vi "Datenauswertung.vi"(7 "Zeit seit dem letzten Aufruf":u32, 8 "Iterationszähler":u8, 11 "Daten aus FPGA-Speicher":u8) -> (0 "Daten für FIFO":u8)   [LabVIEW 2013]
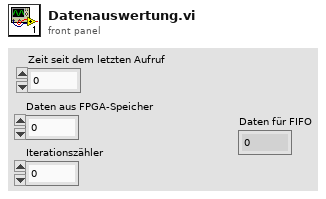
[diagram p1: front panel]
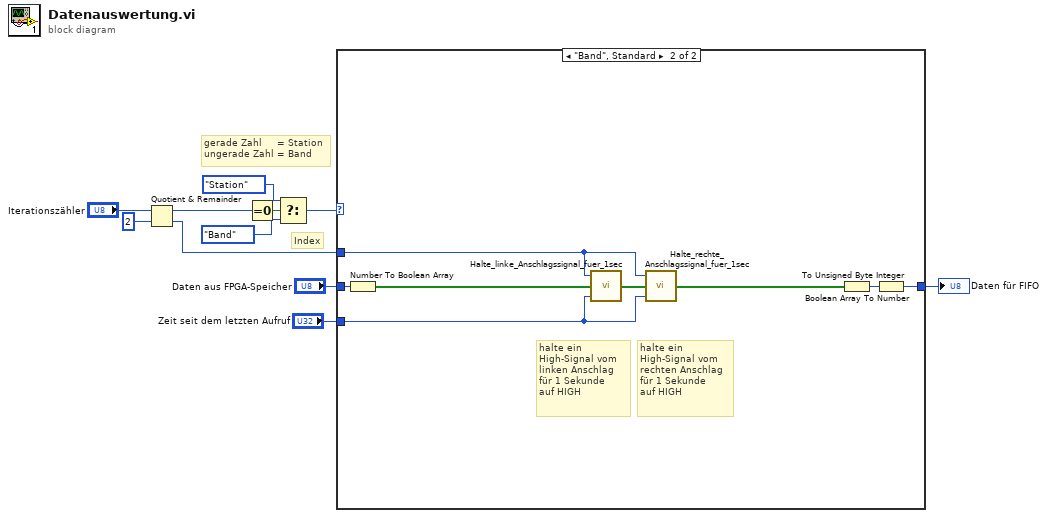
[diagram p0: block diagram]
diagram:
  # "Index"
  # "gerade Zahl     = Station\nungerade Zahl = Band"
  n1 = Quotient & Remainder(x="Iterationszähler", y=u8 2) -> (x-y*floor(x/y)=w5:u8, floor(x/y)=w9:u8)
  n2 = Equal To 0?(x=w5) -> (x = 0?=w4:bool)
  n3 = Select(t=enum16{"Station", "Band"}."Station", s=w4, f=enum16{"Station", "Band"}."Band") -> (s? t:f=w1:enum16{"Station", "Band"})
  n4 = case shown="\"Band\", Standard" w1 {
    tunnel: w9 -> [_ w15]
    tunnel: "Daten aus FPGA-Speicher" -> [w12 w19]
    tunnel: [w12 w13] -> w6
    tunnel: "Zeit seit dem letzten Aufruf" -> [_ w20]
    frame "Station" {
    }
    frame "Band", Default {
      # "halte ein \nHigh-Signal vom\nrechten Anschlag\nfür 1 Sekunde\nauf HIGH"
      # "halte ein \nHigh-Signal vom\nlinken Anschlag\nfür 1 Sekunde\nauf HIGH"
      n5 = Number To Boolean Array(number=w19) -> (Boolean array=w16:bool[])
      n6 = call "Halte_linke_Anschlagssignal_fuer_1sec.vi"("Zeit seit letztem Aufruf"=w20, "Banddaten"=w16, "Band-Index"=w15) -> ("veränderte Banddaten"=w17:bool[])  [unwired: 2 in]
      n7 = call "Halte_rechte_Anschlagssignal_fuer_1sec.vi"("Zeit seit letztem Aufruf"=w20, "Banddaten"=w17, "Band-Index"=w15) -> ("veränderte Banddaten"=w18:bool[])  [unwired: 2 in]
      n8 = Boolean Array To Number(Boolean array=w18) -> (number=w14:u32)
      n9 = To Unsigned Byte Integer(number=w14) -> (unsigned 8bit integer=w13:u8)
    }
  }
  "Daten für FIFO" <- w6
